vi "Log_line.vi"(8 "Data str":string, 9 "résolution":i16, 10 "resu":dbl, 11 "Type":T1=enum."Volt V") -> (3 "message":string)   [LabVIEW 2020]
doc: "Te prepare au format la ligne de log du test\nIN Type [tension, résistance etc]\nIN resu [la valeure du résultat]\nIN Résolution [le nombre de chiffres après la virgule]\nSortie [string]\nex [ohm mOhm;1.7;2]= [R = 1.70 mOhm]"
uses:
  <userlib>/Alex Log/Log_ligne.ctl
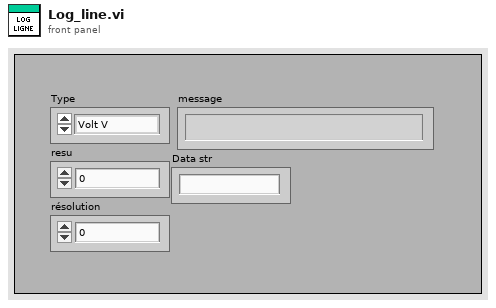
[diagram p1: front panel]
types:
  T1 = typedef "Log_ligne.ctl" = enum16{"Def", "Volt V", "Volt mV", "ohm Ohm", "ohm mOhm", "ohm kOhm", "ohm MOhm", "Opérateur", "EPI", "SN"}
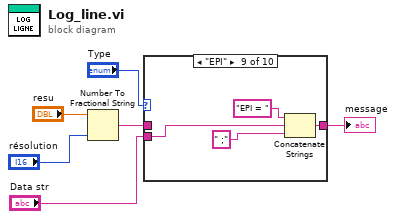
[diagram p0: block diagram]
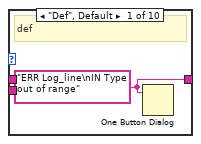
[diagram p2: hidden frame]
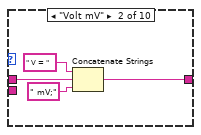
[diagram p3: hidden frame]
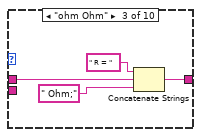
[diagram p4: hidden frame]
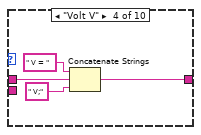
[diagram p5: hidden frame]
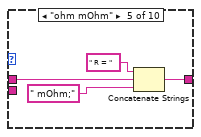
[diagram p6: hidden frame]
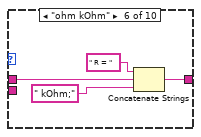
[diagram p7: hidden frame]
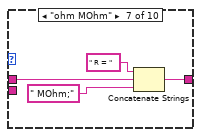
[diagram p8: hidden frame]
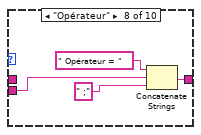
[diagram p9: hidden frame]
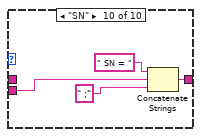
[diagram p10: hidden frame]
diagram:
  n1 = Number To Fractional String(number="resu", precision (6)="résolution") -> (F-format string=w5:string)  [unwired: 2 in]
  n2 = case shown="\"EPI\"" "Type" {
    tunnel: w5 -> [_ w10 w12 w18 w21 w25 w30 _ _ _]
    tunnel: [w7 w8 w13 w16 w20 w24 w28 w33 w36 w40] -> w6
    tunnel: "Data str" -> [_ _ _ _ _ _ _ w32 w37 w41]
    frame "Def", Default {
      w7 = "ERR Log_line\nIN Type out of range" ("message")
      # "def"
      n3 = One Button Dialog(message=w7) -> ()  [unwired: 1 in, 1 out]
    }
    frame "Volt mV" {
      n4 = Concatenate Strings(" V = " ("chaîne"), w10, " mV;" ("chaîne")) -> (w8:string)
    }
    frame "ohm Ohm" {
      n5 = Concatenate Strings(" R = " ("chaîne"), w12, " Ohm;" ("chaîne")) -> (w13:string)
    }
    frame "Volt V" {
      n6 = Concatenate Strings(" V = " ("chaîne"), w18, " V;" ("chaîne")) -> (w16:string)
    }
    frame "ohm mOhm" {
      n7 = Concatenate Strings(" R = " ("chaîne"), w21, " mOhm;" ("chaîne")) -> (w20:string)
    }
    frame "ohm kOhm" {
      n8 = Concatenate Strings(" R = " ("chaîne"), w25, " kOhm;" ("chaîne")) -> (w24:string)
    }
    frame "ohm MOhm" {
      n9 = Concatenate Strings(" R = " ("chaîne"), w30, " MOhm;" ("chaîne")) -> (w28:string)
    }
    frame "Opérateur" {
      n10 = Concatenate Strings(" Opérateur = " ("chaîne"), w32, " ;" ("chaîne")) -> (w33:string)
    }
    frame "EPI" {
      n11 = Concatenate Strings("EPI = " ("chaîne"), w37, " ;" ("chaîne")) -> (w36:string)
    }
    frame "SN" {
      n12 = Concatenate Strings(" SN = " ("chaîne"), w41, " ;" ("chaîne")) -> (w40:string)
    }
  }
  "message" <- w6
